vi "TEST Handle FGV User Event Reference Manager.vi"() -> ()   [LabVIEW 2009]
doc: "This is one of two stub VIs that will be completed in the exercise so that you can test the operation of the FGV User Event Reference Manager.\n\nAAL 9/09"
panel:
  in  "Cancel":bool
  in  "OK":bool
  out "String":string
  out "Data":timestamp
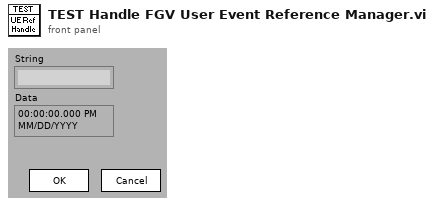
[diagram p1: front panel]
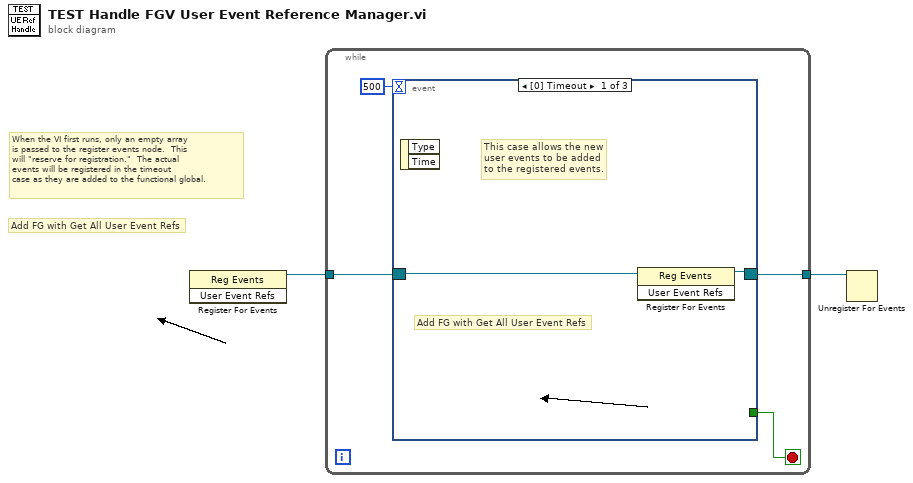
[diagram p0: block diagram]
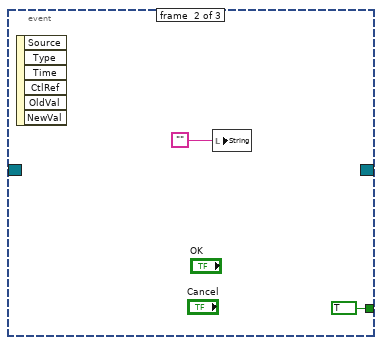
[diagram p2: hidden frame]
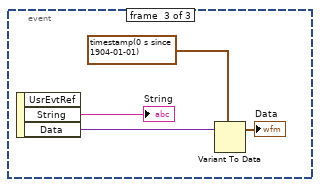
[diagram p3: hidden frame]
diagram:
  # "When the VI first runs, only an empty array\nis passed to the register events node.  This\nwill \"reserve for registration.\"  The actual\nevents will be registered in the timeout\ncase as they are added to the functional global."
  # "Add FG with Get All User Event Refs"
  n1 = register-events() -> (reference out=w2:refnum<event-registration>)  [unwired: 3 in, 1 out]
  n2 = while {
    tunnel: w2 -> [w3]
    tunnel: [w5] -> w1
    stop <- w4 stop-if-true
    n3 = event shown="[0] Timeout" {
      selector: w3 -> [w8 _ _]
      dyn-events: [w7 _ _] -> w5
      timeout: 500 -> [_ _ _]
      tunnel: [_ TRUE ("stop") _] -> w4
      event #0 {
        # "This case allows the new\nuser events to be added\nto the registered events."
        # "Add FG with Get All User Event Refs"
        n4 = event-data() -> ()  [unwired: 3 out]
        n5 = register-events(reference=w8) -> (reference out=w7:refnum<event-registration>)  [unwired: 2 in, 1 out]
      }
      event #1 {
        n6 = event-data() -> ()  [unwired: 7 out]
        n7 = local write "String"("") -> ()
      }
      event #2 {
        n8 = event-data() -> ("String"=→"String":string, "Data"=w12:variant)  [unwired: 2 out]
        n9 = Variant To Data(Variant=w12, type=timestamp(0 s since 1904-01-01)) -> (data=→"Data":timestamp)  [unwired: 1 in, 1 out]
      }
    }
  }
  n10 = Unregister For Events(event registration refnum=w1) -> ()  [unwired: 1 in, 1 out]
